vi "Change file.vi"(8 "Error In":errorcluster, 11 "TDMS-Actor in":refnum<class "TDMS-Actor.lvclass">) -> (0 "Error Out":errorcluster, 3 "TDMS-Actor out":refnum<class "TDMS-Actor.lvclass">)   [LabVIEW 2015, in "BNT_TDMS.lvlib" / "TDMS-Actor.lvclass"]
doc: "Change TDMS file if splitting is requested."
uses:
  TDMS-Actor.lvclass
  TDMS-Actor.lvclass/TDMS-Actor.ctl
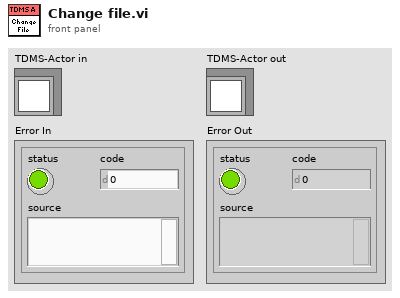
[diagram p1: front panel]
types:
  T1 = enum16{"open", "open or create", "create or replace", "create", "open (read-only)"}
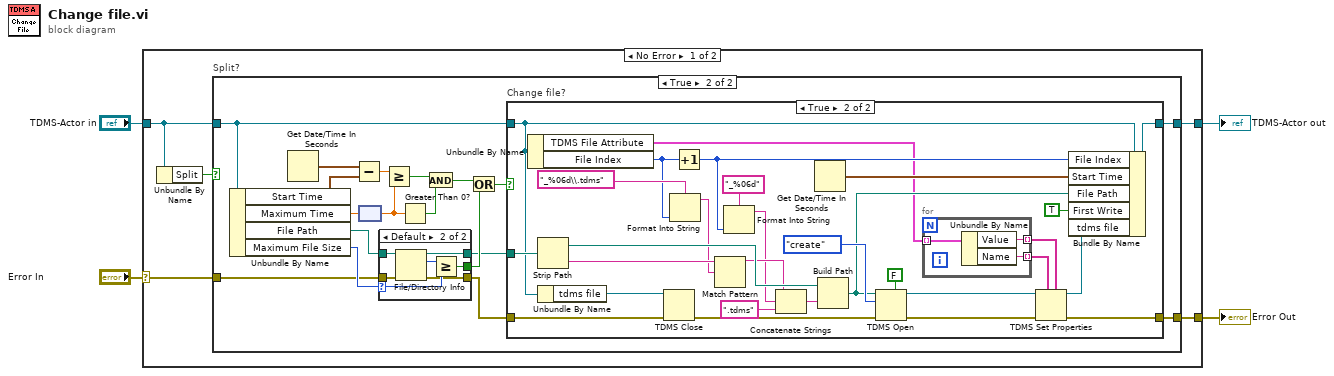
[diagram p0: block diagram]
diagram:
  n1 = case shown="No Error" "Error In" {
    selector: "Error In" -> [w5 w74]
    tunnel: [w6 w74] -> w3
    tunnel: [w7 w73] -> w1
    tunnel: "TDMS-Actor in" -> [w8 w73]
    frame No Error {
      n2 = Unbundle By Name(w8) -> ("Split"=w9:bool)
      n3 = case "Split?" shown="True" w9 {
        tunnel: w8 -> [w11 w17]
        tunnel: [w11 w29] -> w7
        tunnel: [w10 w12] -> w6
        tunnel: w5 -> [w10 w16]
        frame False {
        }
        frame True {
          n4 = Unbundle By Name(w17) -> ("Start Time"=w27:timestamp, "Maximum Time"=w25:dbl[unit], "File Path"=w20:path, "Maximum File Size"=w21:i64)
          n5 = Get Date/Time In Seconds() -> (seconds since 1Jan1904=w28:timestamp)
          n6 = Subtract(x=w28, y=w27) -> (x-y=w26:dbl)
          n7 = node(w25) -> (w24:dbl)
          n8 = case shown="Default" w21 {
            selector: w21 -> [_ w70]
            tunnel: w20 -> [w64 w72]
            tunnel: [_ w69] -> w18
            tunnel: w16 -> [w65 w68]
            tunnel: [w65 w67] -> w13
            tunnel: [w64 w66] -> w14
            frame ..0 {
            }
            frame Default {
              n9 = File/Directory Info(path=w72, error in=w68) -> (path out=w66:path, size=w71:i64, error out=w67:errorcluster)  [unwired: 4 out]
              n10 = Greater Or Equal?(x=w71, y=w70) -> (x >= y?=w69:bool)
            }
          }
          n11 = Greater Or Equal?(x=w26, y=w24) -> (x >= y?=w23:bool)
          n12 = Greater Than 0?(x=w24) -> (x > 0?=w22:bool)
          n13 = And(x=w23, y=w22) -> (x .and. y?=w19:bool)
          n14 = Or(x=w19, y=w18) -> (x .or. y?=w15:bool)
          n15 = case "Change file?" shown="True" w15 {
            tunnel: [w31 w51] -> w29
            tunnel: w17 -> [w31 w44]
            tunnel: w14 -> [_ w53]
            tunnel: w13 -> [w30 w41]
            tunnel: [w30 w38] -> w12
            frame False {
            }
            frame True {
              n16 = Unbundle By Name(w44) -> ("TDMS File Attribute"=w40:cluster{"Name":string, "Value":string}[], "File Index"=w52:i32)
              n17 = Strip Path(path=w53) -> (stripped path=w59:path, name=w58:string)
              n18 = Unbundle By Name(w44) -> ("tdms file"=w43:refnum<k34>)
              n19 = TDMS Close(8:w41, 11:w43) -> (0:w42:errorcluster)  [unwired: 1 out]
              n20 = Format Into String(format string="_%06d\\.tdms", w52) -> (resulting string=w50:string)  [unwired: 2 in, 1 out]
              n21 = Increment(x=w52) -> (x+1=w49:i32)
              n22 = Match Pattern(string=w58, regular expression=w50) -> (before substring=w57:string)  [unwired: 1 in, 3 out]
              n23 = Format Into String(format string="_%06d", w49) -> (resulting string=w47:string)  [unwired: 2 in, 1 out]
              n24 = Concatenate Strings(w57, w47, ".tdms" ("string")) -> (w60:string)
              n25 = Get Date/Time In Seconds() -> (seconds since 1Jan1904=w54:timestamp)
              n26 = Build Path(base path=w59, name or relative path=w60) -> (appended path=w45:path)
              n27 = TDMS Open(5:FALSE ("create index file? (T)"), 8:w42, 10:T1."create" ("operation (0:open)"), 11:w45) -> (0:w39:errorcluster, 3:w34:refnum<k34>)  [unwired: 3 in]
              n28 = for {
                tunnel: w40 -> [w63] mode=indexing
                tunnel: [w62] -> w35 mode=indexing
                tunnel: [w61] -> w36 mode=indexing
                n29 = Unbundle By Name(w63) -> ("Value"=w61:string, "Name"=w62:string)
              }
              n30 = TDMS Set Properties(5:w36, 7:w35, 8:w39, 11:w34) -> (0:w38:errorcluster, 3:w33:refnum<k34>)  [unwired: 2 in, 2 out]
              n31 = Bundle By Name(cluster=w44, "File Index"=w49, "Start Time"=w54, "File Path"=w45, "First Write"=TRUE, "tdms file"=w33) -> (w51:refnum<class "TDMS-Actor.lvclass">)
            }
          }
        }
      }
    }
    frame Error {
    }
  }
  "Error Out" <- w3
  "TDMS-Actor out" <- w1
